vi "TemplateExample.vi"() -> ()   [LabVIEW 2011]
uses:
  Template.ctl
panel:
  in  "Test":T1
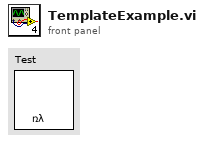
[diagram p1: front panel]
types:
  T1 = typedef "Template.ctl" = bool
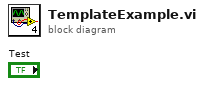
[diagram p0: block diagram]
diagram:
